vi "Check Main Measurement for Instrument Drivers.vi"(0 "instrument containing sub vis in":path[](array[path]), 5 "measurement path":path, 11 "error in":errorcluster) -> (4 "instrument containing sub vis out":path[](array[path]), 15 "error out":errorcluster)   [LabVIEW 2021, in "Multiple Converter.lvlib"]
uses:
  Multiple Converter.lvlib
  Converter Reusables/Converter Reusables.lvlib
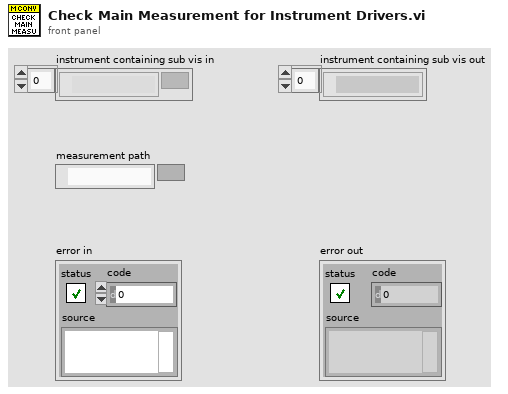
[diagram p1: front panel]
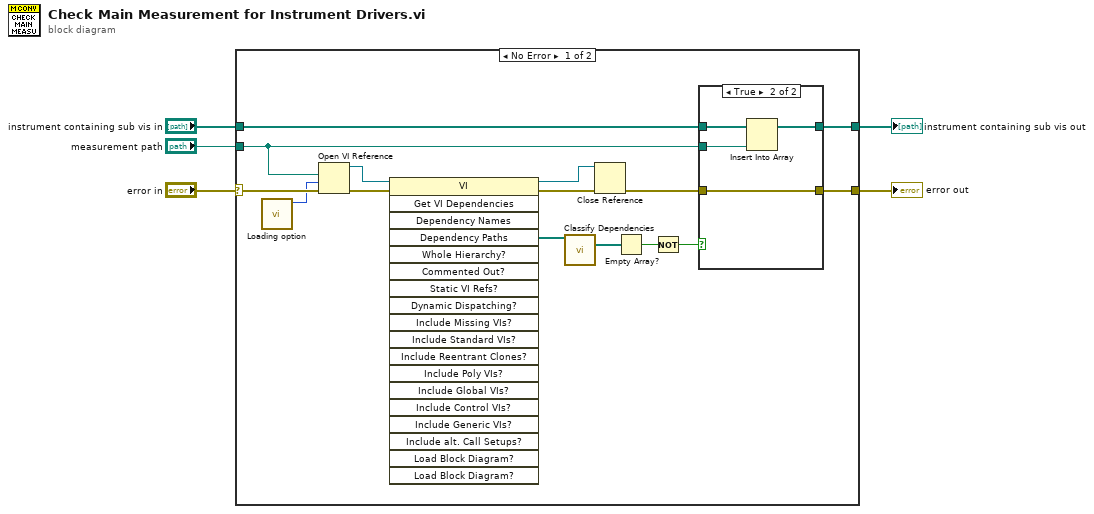
[diagram p0: block diagram]
diagram:
  n1 = case shown="No Error" "error in" {
    selector: "error in" -> [w20 w28]
    tunnel: [w17 w28] -> w5
    tunnel: "measurement path" -> [w13 _]
    tunnel: "instrument containing sub vis in" -> [w19 w27]
    tunnel: [w18 w27] -> w2
    frame No Error {
      n2 = call "Loading option.vi"() -> ("options"=w6:i32)  [unwired: 11 in]
      n3 = Open VI Reference(vi path=w13, options=w6, error in (no error)=w20) -> (vi reference=w12:refnum<vi>, error out=w14:errorcluster)  [unwired: 3 in]
      n4 = invoke class="VI" method="Get VI Dependencies"(reference=w12, error in=w14) -> (reference out=w11:refnum<vi>, error out=w16:errorcluster, "Dependency Paths"=w10:path[])  [unwired: 17 in, 16 out]
      n5 = call "Classify Dependencies.vi"("dependency paths"=w10) -> ("driver vis"=w9:path[])  [unwired: 13 in, 1 out]
      n6 = Close Reference(reference=w11, error in (no error)=w16) -> (error out=w15:errorcluster)
      n7 = Empty Array?(array=w9) -> (empty?=w8:bool)
      n8 = Not(x=w8) -> (.not. x?=w7:bool)
      n9 = case shown="True" w7 {
        tunnel: w15 -> [w22 w23]
        tunnel: w19 -> [w21 w26]
        tunnel: w13 -> [_ w25]
        tunnel: [w21 w24] -> w18
        tunnel: [w22 w23] -> w17
        frame False {
        }
        frame True {
          n10 = Insert Into Array(array=w26, new element=w25) -> (w24:path[])  [unwired: 1 in]
        }
      }
    }
    frame Error {
    }
  }
  "error out" <- w5
  "instrument containing sub vis out" <- w2
